vi "Histogram Window.vi"() -> ()   [LabVIEW 2021, in "Histogram Window.lvlib"]
uses:
  Histogram Window.lvlib
  Histogram Window Q Element v2.ctl
  Histogram Window Q Action v2.ctl
  Graphs/XY Graph/XY Graph Event.ctl
  <vilib>/Utility/miscctls.llb/LVPoint32TypeDef.ctl
  Histogram Updated Plot Info.ctl
  Graphs/Plot Style 3.ctl
  Rich Text Box/Text Formatting.ctl
  Rich Text Box/Text Colors.ctl
  Graphs/XY Graph/XY Graph Mouse Click Event Data.ctl
  Graphs/XY Graph/XY Graph Refnum.ctl
  d1512eee-b5fb-4f95-82d6-c3163d4268d3.vi
  8cc1e088-1b3c-411e-890e-552719ebb6a9.vi
  45187df8-92df-47e4-8ad2-5cf427f9f7d9.vi
  ccf35ae6-8a42-41b8-b330-39459676c0f4.vi
  Graphs/Graphs.lvlib
  Graphs/XY Graph/XY Graph Add-Ons.lvlib
  Notebook/Notebook.lvlib
  Rich Text Box/Rich Text Box.lvlib
  Error/Error.lvlib
panel:
  out "Histogram Graph TipStrip":string caption="Histogram TipStrip"
  out "Histogram Graph":cluster{"Axis":dbl[], "Histogram":dbl[]}[](graph)
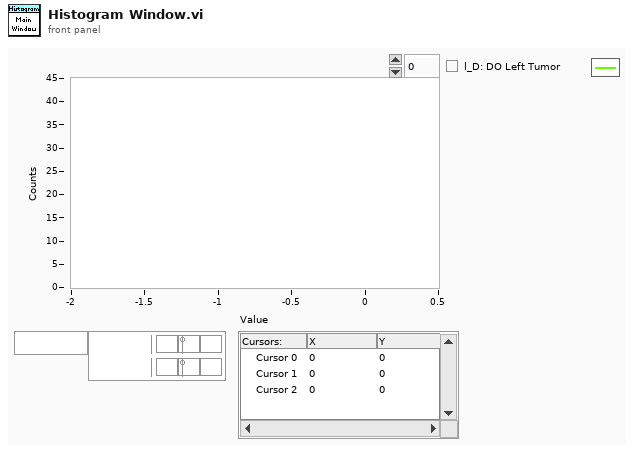
[diagram p1: front panel]
types:
  T1 = typedef "Histogram Window.lvlib/Histogram Window Q Element v2.ctl" = cluster{"Histogram Window Q Action":T2, "Data":variant}
  T2 = typedef "Histogram Window.lvlib/Histogram Window Q Action v2.ctl" = enum16{"Idle", "Initialization", "Generic XY Graph Event", "Add Histogram", "Delete Plot", "Delete Selected Plots", "Clear Graph", "Change Bin Size", "Invert Histogram", "Update Graph", "Plot Fit", "Export XYGraph to Notebook", "Set Last Cursor Style", "Quit"}
  T3 = cluster{"Event Registration Refnum":refnum<event-registration>}
  T4 = typedef "XY Graph Add-Ons.lvlib/XY Graph Event.ctl" = cluster{"Item Tag":string, "XY Graph Refnum":refnum<vi>, "Coords":T5, "Item Path":string}
  T5 = typedef "LVPoint32TypeDef.ctl" = cluster{"Horizontal":i32, "Vertical":i32}
  T6 = typedef "XY Graph Add-Ons.lvlib/XY Graph Mouse Click Event Data.ctl" = cluster{"Multiplot XY Graph":T7, "Mouse Coordinates":T5}
  T7 = typedef "XY Graph Add-Ons.lvlib/XY Graph Refnum.ctl" = refnum<vi>
  T8 = typedef "Histogram Window.lvlib/Histogram Window Internal Variables.ctl" = cluster{"Displayed Histograms":cluster{"Axis":dbl[], "Histogram":dbl[]}[], "Original Bin Histograms":cluster{"Axis":dbl[], "Histogram":dbl[]}[], "Histogram Names":string[]}
  T9 = typedef "Rich Text Box.lvlib/Text Formatting.ctl" = cluster{"Font":string, "Text Color":T10, "Text Background Color":T10, "Text Style":enum16{"Regular", "Bold", "Italic", "Underline", "Strikeout"}, "Font Size (Points)":dbl, "Text Alignment":i32}
  T10 = typedef "Rich Text Box.lvlib/Text Colors.ctl" = enum16{"Unchanged", "Black", "Blue", "Brown", "Gray", "Green", "Orange", "Pink", "Red", "White"}
  T11 = typedef "Histogram Window.lvlib/Histogram Updated Plot Info.ctl" = cluster{"Plot Index":i32, "Plot Name":string, "# Plots":i32, "Plot Style":T12}
  T12 = typedef "Graphs.lvlib/Plot Style 3.ctl" = cluster{"Plot Style":enum16{"unchanged", "Line", "Symbol", "Line + Symbol", "Histogram", "Histogram + Symbol"}, "Histogram Type":enum16{"unchanged", "Left Bound", "Center", "Right Bound"}, "Line Tickness":enum16{"unchanged", "Thin", "1 pixel", "2 pixel", "3 pixel", "4 pixel", "5 pixel"}, "Line Style":enum16{"unchanged", "Plain", "Long Dash", "Short Dash", "Long-Short Dash", "Long-Short-Short Dash"}, "Point Style":enum16{"unchanged", "None", "Empty Circle", "Filled Circle", "Thick Circle", "Dotted Circle", "Empty Square", "Filled Square", "Thick Square", "Dotted Square", "Small Filled Square", "Dot", "Cross", "Tiny Cross", "Large X", "Small x", "Diamond", "Small Empty Square"}, "Line Color":u32, "Point Color":u32, "Anti-aliased":bool, "Line Color Chooser":enum16{"unchanged", "Color Box", "Color List"}, "Point Color Chooser":enum16{"unchanged", "Color Box", "Color List"}, "Line Color List":string, "Point Color List":string}
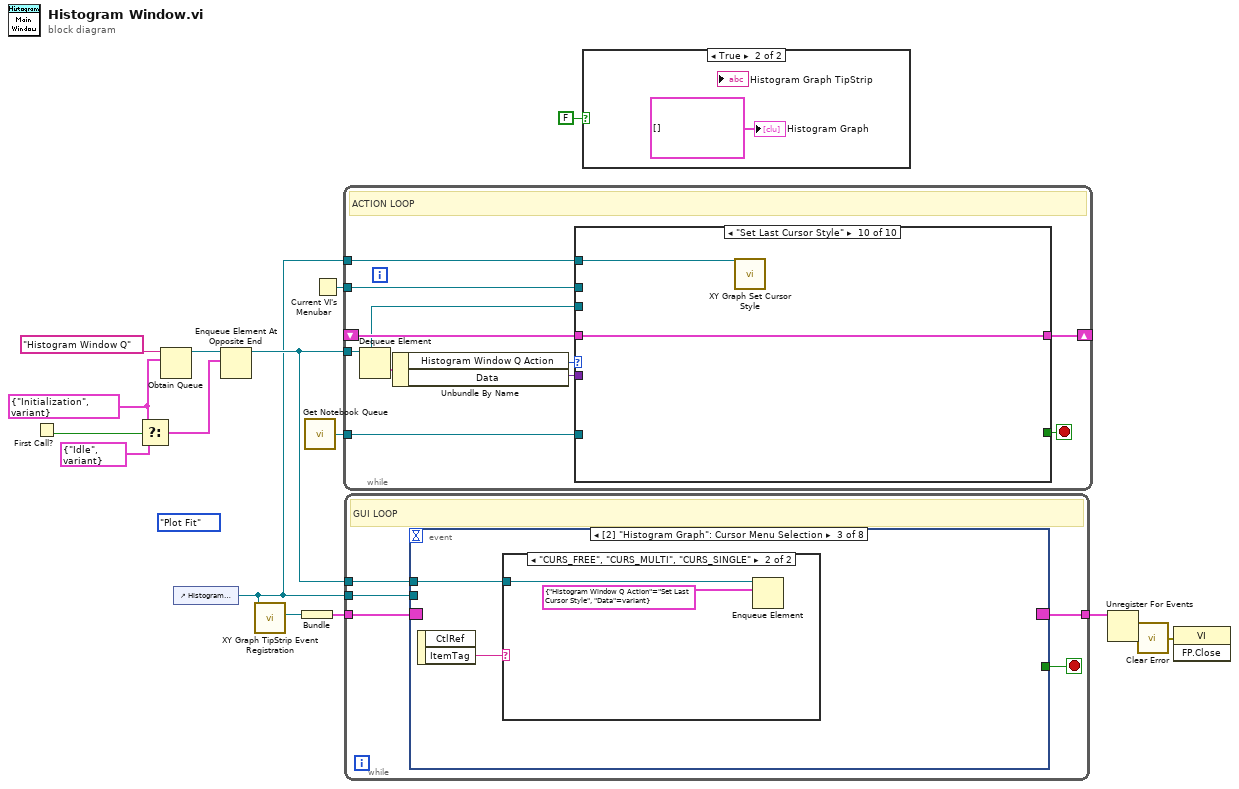
[diagram p0: block diagram]
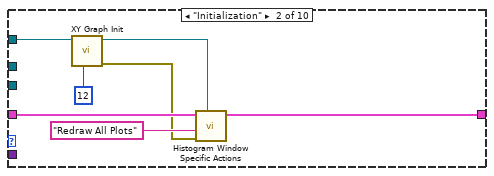
[diagram p4: hidden frame]
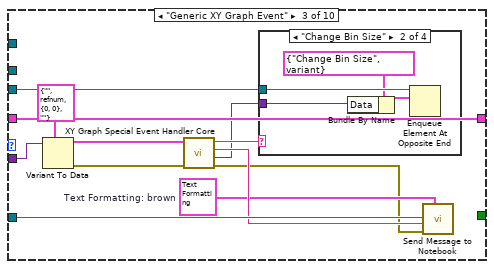
[diagram p5: hidden frame]
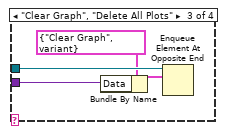
[diagram p7: hidden frame]
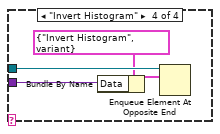
[diagram p8: hidden frame]
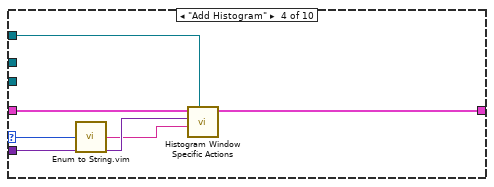
[diagram p9: hidden frame]
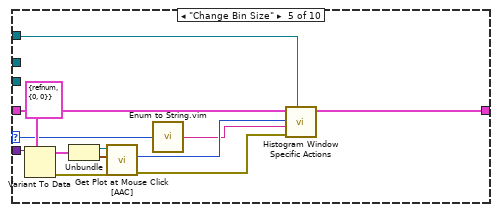
[diagram p10: hidden frame]
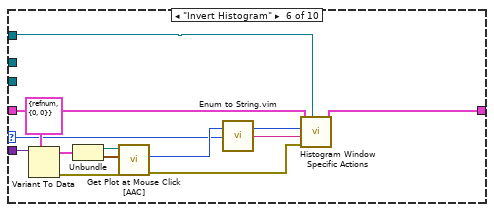
[diagram p11: hidden frame]
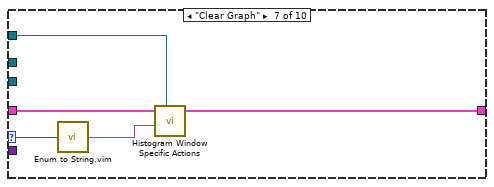
[diagram p12: hidden frame]
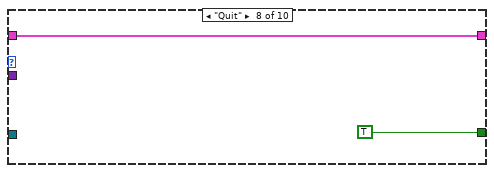
[diagram p13: hidden frame]
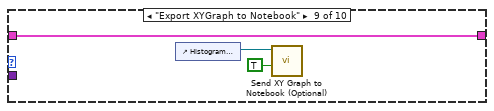
[diagram p14: hidden frame]
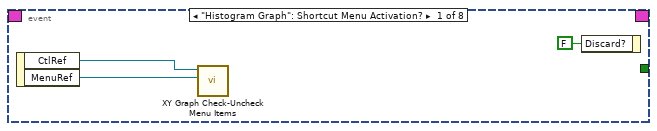
[diagram p15: hidden frame]
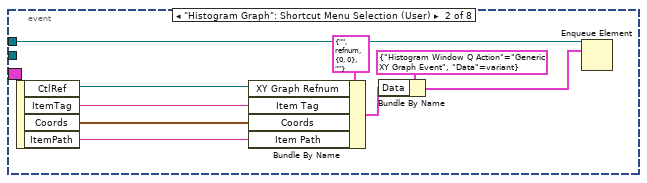
[diagram p16: hidden frame]
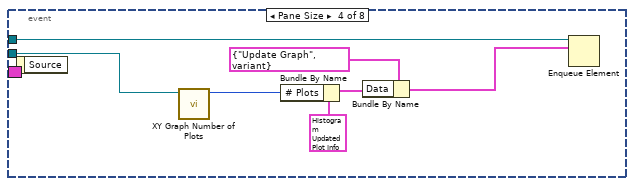
[diagram p18: hidden frame]
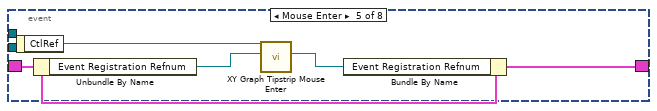
[diagram p19: hidden frame]
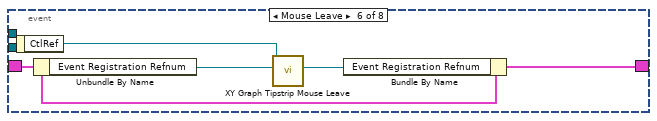
[diagram p20: hidden frame]
diagram:
  (unwired) Histogram_Window_Q_Action_v2."Plot Fit" ("Histogram Window Q Action")
  w5 = T1 {"Histogram Window Q Action"=enum."Initialization", "Data"=variant} ("ALEX TT Histogram Q Element")
  n1 = First Call?() -> (First Call?: T/F=w6:bool)
  n2 = Select(t=w5, s=w6, f=T1 {"Histogram Window Q Action"=enum."Idle", "Data"=variant}) -> (s? t:f=w4:T1)
  n3 = Obtain Queue(name (unnamed)="Histogram Window Q", element data type=w5) -> (queue out=w15:refnum<queue>)  [unwired: 3 in, 2 out]
  n4 = control-ref of="Histogram Graph"() -> (w7:refnum<vi>)
  n5 = Enqueue Element At Opposite End(queue=w15, element=w4) -> (queue out=w14:refnum<queue>)  [unwired: 2 in, 2 out]
  n6 = call "XY Graph TipStrip Event Registration.vi"("XY Graph Refnum"=w7) -> ("Event Registration Refnum"=w10:refnum<event-registration>)  [unwired: 8 in, 2 out]
  n7 = Bundle("Event Registration Refnum"=w10) -> (w12:T3)  [unwired: 1 in]
  n8 = call "Get Notebook Queue.vi"() -> ("Notebook Queue"=w13:refnum<queue>)  [unwired: 9 in]
  n9 = Current VI's Menubar() -> (w8:refnum<k9>)
  n10 = while {
    tunnel: w14 -> [w17]
    tunnel: w13 -> [w22]
    tunnel: w8 -> [w21]
    tunnel: w7 -> [w20]
    shift-right: [w18] -> _
    shift-left: _ -> [w19]
    stop <- w24 stop-if-true
    # "ACTION LOOP"
    n11 = Dequeue Element(queue=w17) -> (element=w26:T1)  [unwired: 2 in, 3 out]
    n12 = Unbundle By Name(w26) -> ("Histogram Window Q Action"=w25:T2, "Data"=w23:variant)
    n13 = case shown="\"Set Last Cursor Style\"" w25 {
      selector: w25 -> [_ _ _ w60 w67 w80 w92 _ _ _]
      tunnel: [_ _ _ _ _ _ _ TRUE _ _] -> w24
      tunnel: w23 -> [_ _ w41 w63 w76 w89 _ _ _ _]
      tunnel: w22 -> [_ _ w43 _ _ _ _ _ _ _]
      tunnel: w21 -> [_ _ _ _ _ _ _ _ _ _]
      tunnel: w20 -> [_ w28 _ w59 w64 w78 w90 _ _ w100]
      tunnel: w19 -> [w27 w32 w38 w62 w68 w81 w94 w95 w97 w101]
      tunnel: [w27 w31 w38 w61 w65 w79 w93 w95 w97 w101] -> w18
      tunnel: w17 -> [_ _ w34 _ _ _ _ _ _ _]
      frame "Idle", Default {
      }
      frame "Initialization" {
        n14 = call "XY Graph Init.vi"("Max Legend Size (8)"=12 ("32bit integer"), "XYGraph in"=w28) -> ("Error Out"=w29:errorcluster)  [unwired: 9 in]
        n15 = call "Histogram Window Specific Actions.vi"("Histogram Graph Refnum"=w28, "Error In"=w29, "Menu Item Tag"="Redraw All Plots", "Histogram Window Internal Variables in"=w32) -> ("Histogram Window Internal Variables out"=w31:T8)  [unwired: 6 in, 1 out]
      }
      frame "Generic XY Graph Event" {
        w39 = T9 {"Font"="Consolas", "Text Color"=enum."Brown", "Text Background Color"=enum."White", "Text Style"=enum."Regular", "Font Size (Points)"=10.0, "Text Alignment"=0}  # Text Formatting: brown
        n16 = Variant To Data(type=T4 {"Item Tag"="", "XY Graph Refnum"=refnum, "Coords"={"Horizontal"=0, "Vertical"=0}, "Item Path"=""} ("XY Graph Event"), Variant=w41) -> (data=w40:T4, error out=w44:errorcluster)  [unwired: 1 in]
        n17 = call "XY Graph Special Event Handler Core.vi"("error in (no error)"=w44, "XY Graph Event"=w40) -> ("error out"=w37:errorcluster, "Data"=w35:variant, "Message"=w42:string, "Menu Item Tag (dup)"=w36:string)  [unwired: 5 in, 1 out]
        n18 = case shown="\"Change Bin Size\"" w36 {
          tunnel: w35 -> [_ w46 w50 w54]
          tunnel: w34 -> [_ w49 w53 w57]
          frame "", Default {
          }
          frame "Change Bin Size" {
            n19 = Bundle By Name(cluster=T1 {"Histogram Window Q Action"=enum."Change Bin Size", "Data"=variant} ("element"), "Data"=w46) -> (w47:T1)
            n20 = Enqueue Element At Opposite End(queue=w49, element=w47) -> ()  [unwired: 2 in, 3 out]
          }
          frame "Clear Graph", "Delete All Plots" {
            n21 = Bundle By Name(cluster=T1 {"Histogram Window Q Action"=enum."Clear Graph", "Data"=variant} ("element"), "Data"=w50) -> (w51:T1)
            n22 = Enqueue Element At Opposite End(queue=w53, element=w51) -> ()  [unwired: 2 in, 3 out]
          }
          frame "Invert Histogram" {
            n23 = Bundle By Name(cluster=T1 {"Histogram Window Q Action"=enum."Invert Histogram", "Data"=variant} ("element"), "Data"=w54) -> (w55:T1)
            n24 = Enqueue Element At Opposite End(queue=w57, element=w55) -> ()  [unwired: 2 in, 3 out]
          }
        }
        n25 = call "Send Message to Notebook.vi"("Text Formatting"=w39, "Error In"=w37, "Message"=w42, "Notebook Queue"=w43) -> ()  [unwired: 4 in, 2 out]
      }
      frame "Add Histogram" {
        n26 = call "Enum to String.vim"("Enum"=w60) -> ("String"=w58:string)
        n27 = call "Histogram Window Specific Actions.vi"("Histogram Graph Refnum"=w59, "Menu Item Tag"=w58, "Data in"=w63, "Histogram Window Internal Variables in"=w62) -> ("Histogram Window Internal Variables out"=w61:T8)  [unwired: 6 in, 1 out]
      }
      frame "Change Bin Size" {
        n28 = Variant To Data(type=T6 {"Multiplot XY Graph"=refnum, "Mouse Coordinates"={"Horizontal"=0, "Vertical"=0}} ("Mouse Click Event Data"), Variant=w76) -> (data=w75:T6, error out=w72:errorcluster)  [unwired: 1 in]
        n29 = Unbundle(w75) -> ("Multiplot XY Graph"=w74:T7, "Mouse Coordinates"=w73:T5)
        n30 = call "Get Plot at Mouse Click [AAC].vi"("error in (no error)"=w72, "Mouse Click Coordinates"=w73, "XYGraph Ref"=w74) -> ("error out"=w70:errorcluster, "Plot at Coordinates"=w71:i32)  [unwired: 2 in, 5 out]
        n31 = call "Enum to String.vim"("Enum"=w67) -> ("String"=w66:string)
        n32 = call "Histogram Window Specific Actions.vi"("Histogram Graph Refnum"=w64, "Error In"=w70, "Menu Item Tag"=w66, "Data in"=w71, "Histogram Window Internal Variables in"=w68) -> ("Histogram Window Internal Variables out"=w65:T8)  [unwired: 5 in, 1 out]
      }
      frame "Invert Histogram" {
        n33 = Variant To Data(type=T6 {"Multiplot XY Graph"=refnum, "Mouse Coordinates"={"Horizontal"=0, "Vertical"=0}} ("Mouse Click Event Data"), Variant=w89) -> (data=w88:T6, error out=w85:errorcluster)  [unwired: 1 in]
        n34 = Unbundle(w88) -> ("Multiplot XY Graph"=w87:T7, "Mouse Coordinates"=w86:T5)
        n35 = call "Get Plot at Mouse Click [AAC].vi"("error in (no error)"=w85, "Mouse Click Coordinates"=w86, "XYGraph Ref"=w87) -> ("error out"=w83:errorcluster, "Plot at Coordinates"=w84:i32)  [unwired: 2 in, 5 out]
        n36 = call "Enum to String.vim"("Enum"=w80) -> ("String"=w77:string)
        n37 = call "Histogram Window Specific Actions.vi"("Histogram Graph Refnum"=w78, "Error In"=w83, "Menu Item Tag"=w77, "Data in"=w84, "Histogram Window Internal Variables in"=w81) -> ("Histogram Window Internal Variables out"=w79:T8)  [unwired: 5 in, 1 out]
      }
      frame "Clear Graph" {
        n38 = call "Enum to String.vim"("Enum"=w92) -> ("String"=w91:string)
        n39 = call "Histogram Window Specific Actions.vi"("Histogram Graph Refnum"=w90, "Menu Item Tag"=w91, "Histogram Window Internal Variables in"=w94) -> ("Histogram Window Internal Variables out"=w93:T8)  [unwired: 7 in, 1 out]
      }
      frame "Quit" {
      }
      frame "Export XYGraph to Notebook" {
        n40 = control-ref of="Histogram Graph"() -> (w99:refnum<vi>)
        n41 = call "Send XY Graph to Notebook (Optional).vi"("Send Graph to Notebook?"=TRUE, "XYGraph in"=w99) -> ()  [unwired: 9 in, 1 out]
      }
      frame "Set Last Cursor Style" {
        n42 = call "XY Graph Set Cursor Style.vi"("XYGraph Refnum"=w100) -> ()  [unwired: 9 in, 2 out]
      }
    }
  }
  n43 = while {
    tunnel: w14 -> [w105]
    tunnel: w12 -> [w103]
    tunnel: [w104] -> w9
    tunnel: w7 -> [w102]
    stop <- w106 stop-if-true
    # "GUI LOOP"
    n44 = event shown="[2] \"Histogram Graph\": Cursor Menu Selection" {
      selector: w103 -> [_ _ _ _ w134 w139 w141 _]
      dyn-events: [_ _ _ _ w133 w138 w141 _] -> w104
      timeout: _ -> [_ _ _ _ _ _ _ _]
      tunnel: [_ _ _ _ _ _ _ w146] -> w106
      tunnel: w105 -> [_ w115 w119 w129 _ _ _ w145]
      tunnel: w102 -> [_ _ _ w123 _ _ _ _]
      event "Histogram Graph": Shortcut Menu Activation? {
        n45 = event-data() -> ("CtlRef"=w107:refnum<vi>, "MenuRef"=w108:refnum<k9>)  [unwired: 1 in]
        n46 = call "XY Graph Check-Uncheck Menu Items.vi"("Menu in"=w108, "XY Graph Refnum"=w107) -> ()  [unwired: 6 in, 4 out]
        n47 = event-data("Discard?"=FALSE) -> ()  [unwired: 1 in, 1 out]
      }
      event "Histogram Graph": Shortcut Menu Selection (User) {
        n48 = event-data() -> ("CtlRef"=w118:refnum<vi>, "ItemTag"=w117:string, "Coords"=w116:T5, "ItemPath"=w114:string)  [unwired: 1 in]
        n49 = Bundle By Name(cluster=T4 {"Item Tag"="", "XY Graph Refnum"=refnum, "Coords"={"Horizontal"=0, "Vertical"=0}, "Item Path"=""} ("XY Graph Event"), "XY Graph Refnum"=w118, "Item Tag"=w117, "Coords"=w116, "Item Path"=w114) -> (w113:T4)
        n50 = Bundle By Name(cluster=T1 {"Histogram Window Q Action"=enum."Generic XY Graph Event", "Data"=variant} ("element"), "Data"=w113) -> (w110:T1)
        n51 = Enqueue Element(queue=w115, element=w110) -> ()  [unwired: 2 in, 3 out]
      }
      event "Histogram Graph": event #0x4e {
        n52 = event-data() -> ("ItemTag"=w120:string)  [unwired: 1 in, 1 out]
        n53 = case shown="\"CURS_FREE\", \"CURS_MULTI\", \"CURS_SINGLE\"" w120 {
          tunnel: w119 -> [_ w122]
          frame "", Default {
          }
          frame "CURS_FREE", "CURS_MULTI", "CURS_SINGLE" {
            n54 = Enqueue Element(queue=w122, element=T1 {"Histogram Window Q Action"=enum."Set Last Cursor Style", "Data"=variant}) -> ()  [unwired: 2 in, 3 out]
          }
        }
      }
      event Pane Size {
        n55 = event-data() -> ()  [unwired: 1 in, 1 out]
        n56 = call "XY Graph Number of Plots.vi"("XYGraph in"=w123) -> ("# Plots"=w124:i32)  [unwired: 9 in, 1 out]
        n57 = Bundle By Name(cluster=T11 {"Plot Index"=-1, "Plot Name"="", "# Plots"=0, "Plot Style"={"Plot Style"=enum."Histogram + Symbol", "Histogram Type"=enum."Right Bound", "Line Tickness"=enum."unchanged", "Line Style"=enum."unchanged", "Point Style"=enum."unchanged", "Line Color"=0, "Point Color"=0, "Anti-aliased"=FALSE, "Line Color Chooser"=enum."unchanged", "Point Color Chooser"=enum."unchanged", "Line Color List"="", "Point Color List"=""}} ("Updated Plot Info"), "# Plots"=w124) -> (w125:T11)
        n58 = Bundle By Name(cluster=T1 {"Histogram Window Q Action"=enum."Update Graph", "Data"=variant} ("element"), "Data"=w125) -> (w127:T1)
        n59 = Enqueue Element(queue=w129, element=w127) -> ()  [unwired: 2 in, 3 out]
      }
      event Mouse Enter {
        n60 = event-data() -> ("CtlRef"=w132:refnum<vi>)  [unwired: 1 in]
        n61 = Unbundle By Name(w134) -> ("Event Registration Refnum"=w131:refnum<event-registration>)
        n62 = call "XY Graph Tipstrip Mouse Enter.vi"("Event Registration Refnum"=w131, "XY Graph Refnum"=w132) -> ("Event Registration Refnum"=w130:refnum<event-registration>)  [unwired: 8 in, 1 out]
        n63 = Bundle By Name(cluster=w134, "Event Registration Refnum"=w130) -> (w133:T3)
      }
      event Mouse Leave {
        n64 = event-data() -> ("CtlRef"=w137:refnum<vi>)  [unwired: 1 in]
        n65 = Unbundle By Name(w139) -> ("Event Registration Refnum"=w136:refnum<event-registration>)
        n66 = call "XY Graph Tipstrip Mouse Leave.vi"("Event Registration Refnum"=w136, "XY Graph Refnum"=w137) -> ("Event Registration Refnum"=w135:refnum<event-registration>)  [unwired: 8 in, 1 out]
        n67 = Bundle By Name(cluster=w139, "Event Registration Refnum"=w135) -> (w138:T3)
      }
      event Mouse Move {
        n68 = event-data() -> ("CtlRef"=w143:refnum<vi>, "Coords"=w142:T5)  [unwired: 1 in]
        n69 = call "XY Graph TipStrip Mouse Move.vi"("Coords"=w142, "XY Graph Refnum"=w143) -> ("Error Out"=w140:errorcluster)  [unwired: 7 in, 2 out]
        n70 = call <vilib>:"Clear Errors.vi"("error in (no error)"=w140) -> ()  [unwired: 5 in, 2 out]
      }
      event Panel Close? {
        w146 = TRUE
        n71 = event-data() -> ()  [unwired: 1 in, 3 out]
        n72 = Enqueue Element(queue=w145, element=T1 {"Histogram Window Q Action"=enum."Quit", "Data"=variant} ("ALEX TT Histogram Q Element")) -> ()  [unwired: 2 in, 3 out]
        n73 = event-data("Discard?"=w146) -> ()  [unwired: 1 in, 1 out]
      }
    }
  }
  n74 = case shown="True" FALSE {
    frame False {
    }
    frame True {
      "Histogram Graph" <- cluster{"Axis":dbl[], "Histogram":dbl[]}[] [] ("Histogram Graph")
    }
  }
  n75 = Unregister For Events(event registration refnum=w9) -> (error out=w2:errorcluster)  [unwired: 1 in]
  n76 = call "Clear Error.vi"("Error In"=w2) -> ("no Error Out"=w1:errorcluster)  [unwired: 8 in]
  n77 = invoke class="VI" method="FP.Close"(error in=w1) -> ()  [unwired: 2 in, 3 out]
